vi "trash_Check Read.vi"(8 "error in (no error)":errorcluster, 11 "CIFChannels in":refnum<class "CIFChannels.lvclass">) -> (0 "error out":errorcluster, 2 "Not Connected":bool, 3 "CIFChannels out":refnum<class "CIFChannels.lvclass">)   [LabVIEW 2021]
uses:
  CIFChannels.lvclass
  CIFChannels.lvclass/CIFChannels.ctl
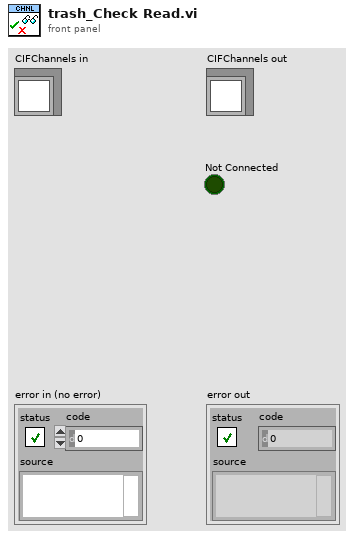
[diagram p1: front panel]
types:
  T1 = typedef "CIFChannels.lvclass/Channel State.ctl" = enum16{"Creating", "Disconnected", "Connecting", "Connected", "Destroying"}
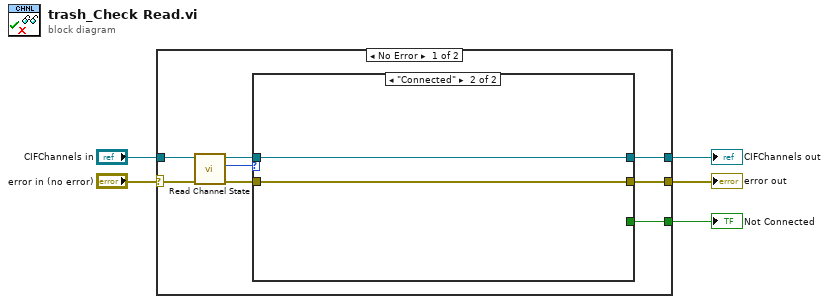
[diagram p0: block diagram]
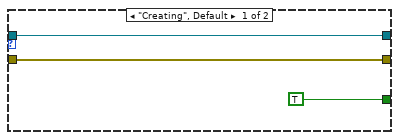
[diagram p2: hidden frame]
diagram:
  n1 = case shown="No Error" "error in (no error)" {
    selector: "error in (no error)" -> [w12 w20]
    tunnel: [w6 w20] -> w4
    tunnel: [w9 w19] -> w2
    tunnel: "CIFChannels in" -> [w13 w19]
    tunnel: [w7 _] -> w1
    frame No Error {
      n2 = call "Read Channel State.vi"("error in (no error)"=w12, "CIFChannels in"=w13) -> ("error out"=w8:errorcluster, "Channel State"=w11:T1, "CIFChannels out"=w10:refnum<class "CIFChannels.lvclass">)  [unwired: 7 in]
      n3 = case shown="\"Connected\"" w11 {
        tunnel: w10 -> [w14 w18]
        tunnel: [w14 w18] -> w9
        tunnel: w8 -> [w15 w17]
        tunnel: [w15 w17] -> w6
        tunnel: [TRUE _] -> w7
        frame "Creating", Default {
        }
        frame "Connected" {
        }
      }
    }
    frame Error {
    }
  }
  "error out" <- w4
  "CIFChannels out" <- w2
  "Not Connected" <- w1
